vi "AddParametersToSweepResults.vi"(8 "error in (no error)":errorcluster, 9 "SweepResults [i]":T1, 10 "AO":waveform(dbl)[](array[waveform]), 11 "Lockin.DAQ":refnum<class "Instrument.DAQ.lvclass">) -> (0 "error out":errorcluster, 1 "SweepResults [i] out":T1, 3 "Lockin.DAQ out":refnum<class "Instrument.DAQ.lvclass">)   [LabVIEW 2019, in "Instrument.DAQ.lvclass"]
uses:
  Instrument.DAQ.lvclass
  <vilib>/measure/NI_MAPro.lvlib
  <vilib>/measure/maresamp.llb/Resample Waveform (single shot).vi
  Typedefs/SweepResults--Cluster.ctl
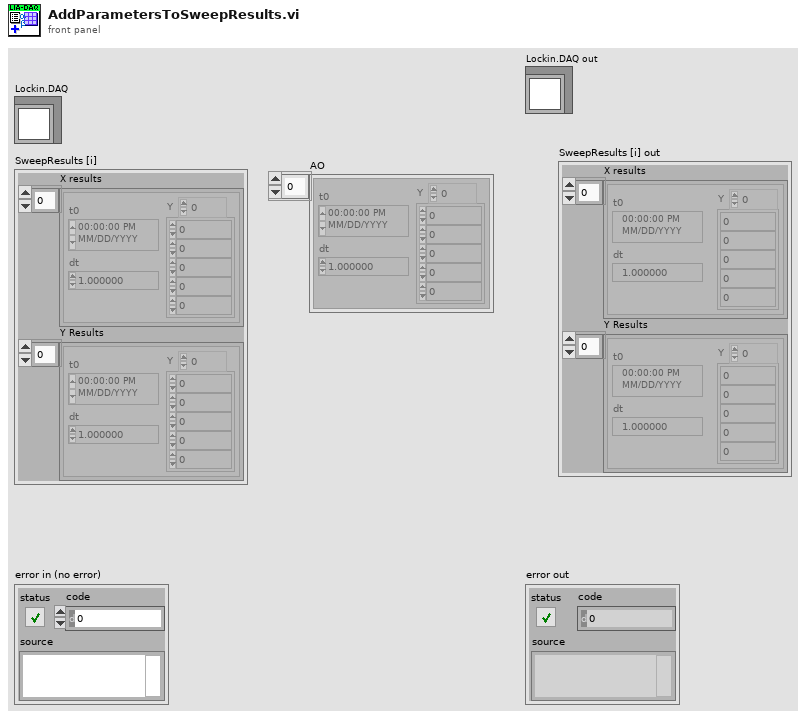
[diagram p1: front panel]
types:
  T1 = typedef "Instrument.DAQ.lvclass/SweepResults--Cluster.ctl" = cluster{"X results":waveform(dbl)[], "Y Results":waveform(dbl)[]}
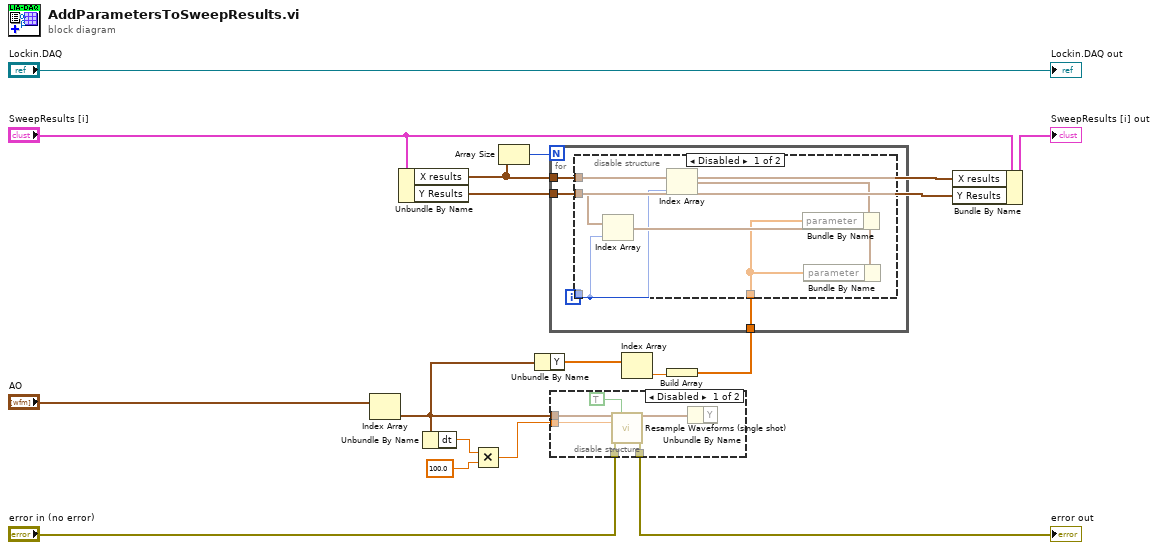
[diagram p0: block diagram]
diagram:
  n1 = Index Array(array="AO") -> (element=w6:waveform(dbl))  [unwired: 1 in]
  n2 = Unbundle By Name("SweepResults [i]") -> ("X results"=w2:waveform(dbl)[], "Y Results"=w1:waveform(dbl)[])
  n3 = Unbundle By Name(w6) -> ("dt"=w8:dbl)
  n4 = Multiply(x=w8, y=100.0) -> (x*y=w7:dbl)
  n5 = Array Size(array=w2) -> (size(s)=w16:i32)
  n6 = Unbundle By Name(w6) -> ("Y"=w5:dbl[])
  n7 = disable-structure shown="Disabled" {
    disable-tunnel: "error in (no error)" -> [w21 w23]
    disable-tunnel: [w20 w23] -> w10
    disable-tunnel: w7 -> [w18 _]
    disable-tunnel: w6 -> [w17 _]
    frame Disabled {
      n8 = call-poly <vilib>:"Resample Waveforms (single shot).vi"("waveform in"=w17, "open interval? (F)"=TRUE, "dt"=w18, "error in (no error)"=w21) -> ("resampled waveform out"=w22:waveform(dbl), "error out"=w20:errorcluster)  [unwired: 8 in, 2 out]
      n9 = Unbundle By Name(w22) -> ()  [unwired: 1 out]
    }
    frame Enabled {
    }
  }
  "error out" <- w10
  n10 = Index Array(array=w5) -> (element=w4:dbl)  [unwired: 1 in]
  n11 = Build Array(w4) -> (w3:dbl[])
  n12 = for {
    N: w16 -> [_]
    tunnel: w2 -> [w27]
    tunnel: w1 -> [w26]
    tunnel: w3 -> [w25]
    i -> [w24]
    n13 = disable-structure shown="Disabled" {
      disable-tunnel: w27 -> [w34 _]
      disable-tunnel: w26 -> [w33 _]
      disable-tunnel: w25 -> [w29 _]
      disable-tunnel: w24 -> [w28 _]
      frame Disabled {
        n14 = Index Array(array=w33, index=w28) -> (element=w31:waveform(dbl))
        n15 = Index Array(array=w34, index=w28) -> (element=w30:waveform(dbl))
        n16 = Bundle By Name(cluster=w30, "parameter"=w29) -> ()  [unwired: 1 out]
        n17 = Bundle By Name(cluster=w31, "parameter"=w29) -> (w32:cluster{})
      }
      frame Enabled {
      }
    }
  }
  n18 = Bundle By Name(cluster="SweepResults [i]", "X results"=w2, "Y Results"=w1) -> (→"SweepResults [i] out":T1)
  "Lockin.DAQ out" <- "Lockin.DAQ"
